vi "Get Time Date Display String.vi"(8 "error in \n(no error)":errorcluster, 11 "test\n results in":refnum<class "Test Results Base Class.lvclass">) -> (0 "error out":errorcluster, 2 "concatenated string":string, 3 "test results out":refnum<class "Test Results Base Class.lvclass">)   [LabVIEW 2020, in "Test Results Base Class.lvclass"]
doc: "This VI is an example of a private member VI. Only VIs within the same class can call this VI."
uses:
  Test Results Base Class.lvclass
  Test Results Base Class.lvclass/Test Results Base Class.ctl
panel:
  # "This VI is an example of a private member VI of a LabVIEW class.\nOnly VIs within the same class can call this VI."
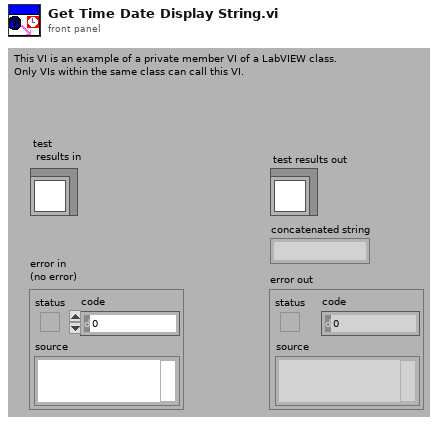
[diagram p1: front panel]
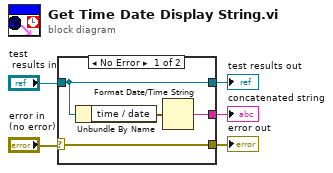
[diagram p0: block diagram]
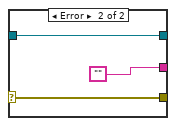
[diagram p2: hidden frame]
diagram:
  n1 = case shown="No Error" "error in \n(no error)" {
    selector: "error in \n(no error)" -> [w9 w12]
    tunnel: [w9 w12] -> w4
    tunnel: "test\n results in" -> [w8 w11]
    tunnel: [w8 w11] -> w2
    tunnel: [w6 "" ("Empty String Constant")] -> w1
    frame No Error {
      n2 = Unbundle By Name(w8) -> ("time / date"=w7:timestamp)
      n3 = Format Date/Time String(seconds (now)=w7) -> (date/time string=w6:string)  [unwired: 2 in]
    }
    frame Error {
    }
  }
  "test results out" <- w2
  "error out" <- w4
  "concatenated string" <- w1
